vi "SETI_FPGA Interface.vi"() -> ()   [LabVIEW 2015]
uses:
  <vilib>/rvi/interface/nirviMethod/nirviMethod.xnode
  <vilib>/rvi/interface/nirviReadWriteControl/nirviReadWriteControl.xnode
  <vilib>/rvi/interface/nirviOpenFPGA/nirviOpenFPGA.xnode
  <vilib>/rvi/interface/nirviCloseFPGA/nirviCloseFPGA.xnode
  <vilib>/Utility/error.llb/Error Cluster From Error Code.vi
  <vilib>/rvi/interface/Simulation/niFpgaSimulationCallBeginRW.vi
  <vilib>/rvi/errors/niLvFpgaAdjustHostInterfaceError.vi
  <vilib>/rvi/errors/niLvFpgaMergeErrorWithErrorCode.vi
  <vilib>/FPGAPlugInAG/Dynamic/niLvFpga_ReadFifo_Dynamic.vi
  <vilib>/FPGAPlugInAG/Dynamic/niLvFpga_ConfigureFifo_Dynamic.vi
  FPGA Target/Old/SETI_Host_Interface.vi
  NiFpgaLv.dll
  <vilib>/FPGAPlugInAG/Dynamic/niLvFpga_WriteFifo_Dynamic.vi
  <vilib>/FPGAPlugInAG/Dynamic/niLvFpga_Close_Dynamic.vi
  <vilib>/rvi/interface/RandomDataEmulation/nirviRandomDataOpen.vi
  <vilib>/rvi/interface/common/niFpgaCacheSessionInfoDynamic.vi
panel:
  in  "Inputs":i32=2500
  out "Ok?":bool
  out "FPGA Loop Count":i32
  out "State":enum16{"Idle", "Start", "Process", "Stop"}(ring)
  out "Total":u64
  out "Count":i32
  out "Number of Data Points":i16
  out "Start":bool
  out "Loop Count":i32
  out "Elements Remaining":u32
  out "Output":u64[](array[numeric])
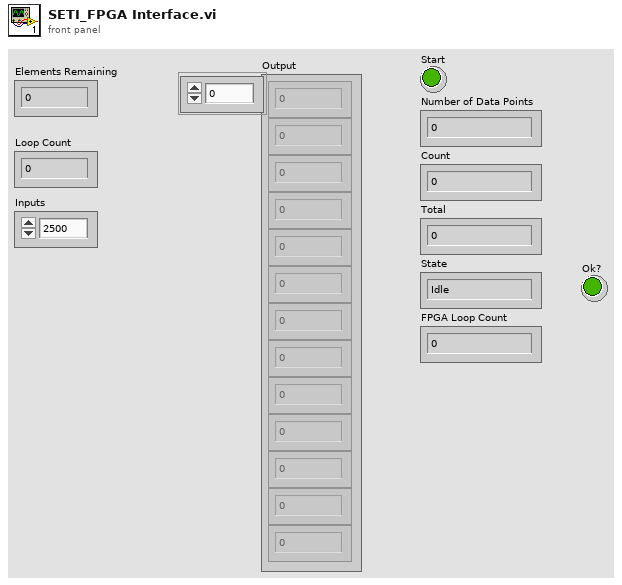
[diagram p1: front panel]
types:
  T1 = enum16{"Idle", "GetNumPoints", "GetChirpRate", "Process", "Stop"}
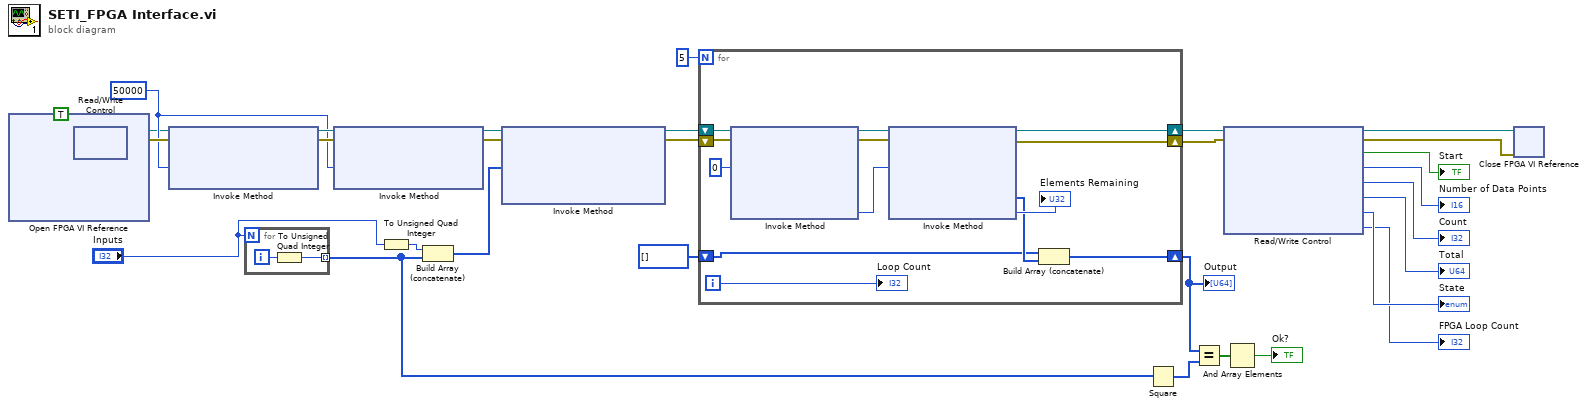
[diagram p0: block diagram]
diagram:
  w13 = u32 50000 ("Requested Depth")
  n1 = xnode "Open FPGA VI Reference"() -> ("FPGA VI Reference Out"=w32:refnum<k20>, "error out"=w31:errorcluster)  [unwired: 2 in]
  n2 = xnode "Read/Write Control"("FPGA VI Reference In"=w32, "error in"=w31, "Start"=TRUE ("Boolean")) -> ("FPGA VI Reference Out"=w9:refnum<k20>, "error out"=w16:errorcluster)
  n3 = xnode "Invoke Method"("FPGA VI Reference In"=w9, "error in"=w16, "Requested Depth"=w13) -> ("FPGA VI Reference Out"=w15:refnum<k20>, "error out"=w14:errorcluster)  [unwired: 1 out]
  n4 = for {
    N: "Inputs" -> [_]
    tunnel: [w33] -> w4 mode=indexing
    i -> [w34]
    n5 = To Unsigned Quad Integer(1:w34) -> (0:w33:u64)
  }
  n6 = xnode "Invoke Method"("FPGA VI Reference In"=w15, "error in"=w14, "Requested Depth"=w13) -> ("FPGA VI Reference Out"=w12:refnum<k20>, "error out"=w11:errorcluster)  [unwired: 1 out]
  n7 = To Unsigned Quad Integer(1:"Inputs") -> (0:w6:u64)
  n8 = Build Array (concatenate)(w6, w4) -> (w8:u64[])
  n9 = xnode "Invoke Method"("FPGA VI Reference In"=w12, "error in"=w11, "Data"=w8) -> ("FPGA VI Reference Out"=w29:refnum<k20>, "error out"=w28:errorcluster)  [unwired: 1 in, 1 out]
  n10 = for {
    N: 5 -> [_]
    shift-right: [w35] -> w5
    shift-left: u64[] [] -> [w45]
    shift-right: [w43] -> w25
    shift-left: w29 -> [w41]
    shift-right: [w42] -> w24
    shift-left: w28 -> [w40]
    i -> [w44]
    n11 = xnode "Invoke Method"("FPGA VI Reference In"=w41, "error in"=w40, "Number of Elements"=u32 0) -> ("FPGA VI Reference Out"=w39:refnum<k20>, "error out"=w38:errorcluster, "Elements Remaining"=w36:u32)  [unwired: 1 in, 1 out]
    n12 = xnode "Invoke Method"("FPGA VI Reference In"=w39, "error in"=w38, "Number of Elements"=w36) -> ("FPGA VI Reference Out"=w43:refnum<k20>, "error out"=w42:errorcluster, "Data"=w46:u64[], "Elements Remaining"=→"Elements Remaining":u32)  [unwired: 1 in]
    n13 = Build Array (concatenate)(w45, w46) -> (w35:u64[])
    "Loop Count" <- w44
  }
  "Output" <- w5
  n14 = Square(x=w4) -> (x^2=w3:u64[])
  n15 = Equal?(x=w5, y=w3) -> (x = y?=w2:bool[])
  n16 = xnode "Read/Write Control"("FPGA VI Reference In"=w25, "error in"=w24) -> ("FPGA VI Reference Out"=w19:refnum<k20>, "error out"=w18:errorcluster, "Start"=→"Start":bool, "Number of Data Points"=→"Number of Data Points":i16, "Count"=→"Count":i32, "Total"=→"Total":u64, "State"=→"State":T1, "FPGA Loop Count"=→"FPGA Loop Count":i32)
  n17 = And Array Elements(Boolean array=w2) -> (logical AND=→"Ok?":bool)
  n18 = xnode "Close FPGA VI Reference"("FPGA VI Reference In"=w19, "error in"=w18) -> ()  [unwired: 1 out]
